vi "00E0.vi"(11 "Variables and Memory in":T1 {"GFX" format="%02x"}) -> (3 "Variables and Memory out":T1 {"GFX" format="%02x"})   [LabVIEW 2021]
uses:
  Controls/ClusterF.ctl
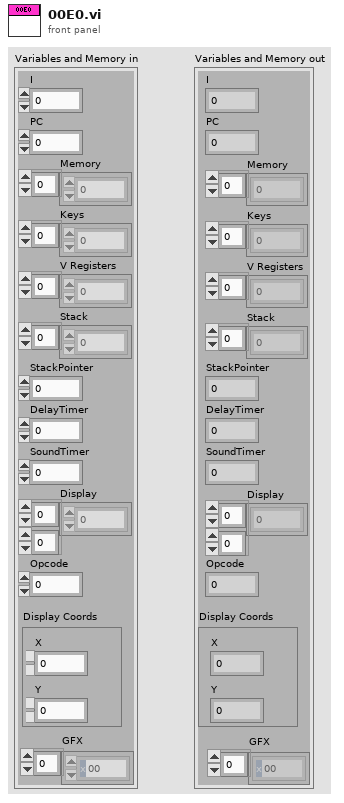
[diagram p1: front panel]
types:
  T1 = typedef "ClusterF.ctl" = cluster{"I":u16, "PC":u16, "Memory":u8[], "Keys":u8[], "V Registers":u8[], "Stack":u16[], "StackPointer":u16, "DelayTimer":u8, "SoundTimer":u8, "Display":u8[][], "Opcode":u16, "Display Coords":cluster{"X":u8, "Y":u8}, "GFX":u8[]}
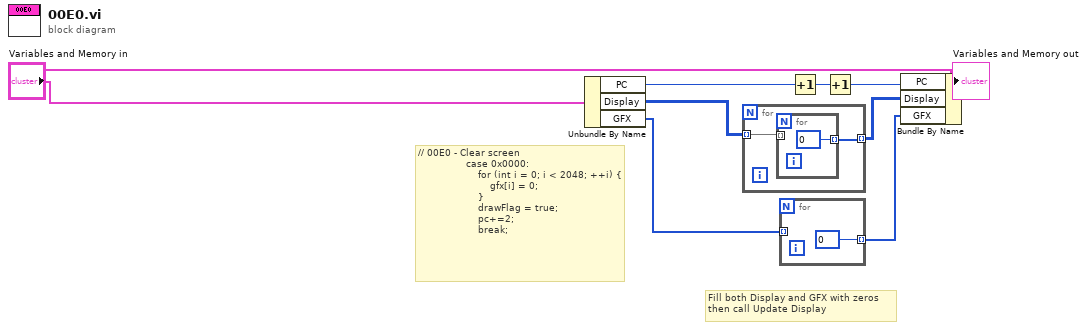
[diagram p0: block diagram]
diagram:
  # "Fill both Display and GFX with zeros\nthen call Update Display"
  # "// 00E0 - Clear screen\n                case 0x0000:\n                    for (int i = 0; i < 2048; ++i) {\n                        gfx[i] = 0;\n                    }\n                    drawFlag = true;\n                    pc+=2;\n                    break;"
  n1 = Unbundle By Name("Variables and Memory in") -> ("PC"=w2:u16, "Display"=w6:u8[][], "GFX"=w8:u8[])
  n2 = for {
    tunnel: w6 -> [w11] mode=indexing
    tunnel: [w10] -> w7 mode=indexing
    n3 = for {
      tunnel: w11 -> [_] mode=indexing
      tunnel: [u8 0] -> w10 mode=indexing
    }
  }
  n4 = for {
    tunnel: w8 -> [_] mode=indexing
    tunnel: [u8 0] -> w9 mode=indexing
  }
  n5 = Increment(x=w2) -> (x+1=w1:u16)
  n6 = Increment(x=w1) -> (x+1=w5:u16)
  n7 = Bundle By Name(cluster="Variables and Memory in", "PC"=w5, "Display"=w7, "GFX"=w9) -> (→"Variables and Memory out":T1)
